vi "Build move command.vi"(8 "error in (no error)":errorcluster, 10 "Command":T1 {"Step style motor 2" items=["", "Single", "Double", "Interleave", "Microstep"]; "Step style motor 1" items=["", "Single", "Double", "Interleave", "Microstep"]; "Direction motor 2" items=["", "Forward", "Backward"]; "Direction motor 1" items=["", "Forward", "Backward"]; "Action" items=["", "Initialize", "Move"]}, 11 "VISA Refnum in":refnum<visa-resource-name>) -> (0 "error out":errorcluster, 2 "String":string, 3 "VISA Refnum out":refnum<visa-resource-name>)   [LabVIEW 2020, in "Arduino-Adafruit stepper.lvlib"]
uses:
  Arduino-Adafruit stepper.lvlib
  Move motor parameters--cluster.ctl
  Motor direction.ctl
  Step style.ctl
  <vilib>/Instr/_visa.llb/VISA Flush IO Buffer Mask.ctl
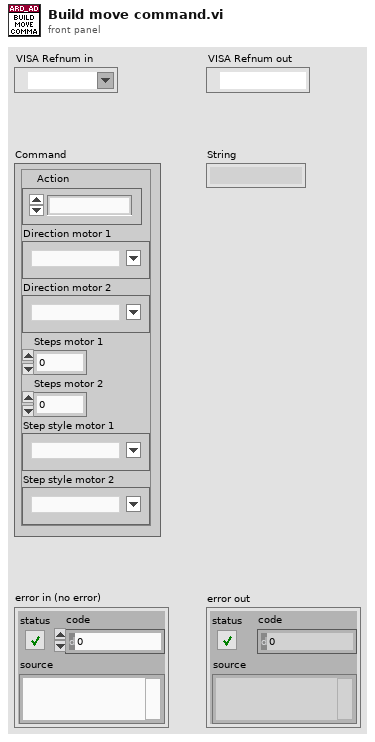
[diagram p1: front panel]
types:
  T1 = typedef "Arduino-Adafruit stepper.lvlib/Move motor parameters--cluster.ctl" = cluster{"Action":u8, "Direction motor 1":T2, "Direction motor 2":T2, "Steps motor 1":u16, "Steps motor 2":u16, "Step style motor 1":T3, "Step style motor 2":T3}
  T2 = typedef "Arduino-Adafruit stepper.lvlib/Motor direction.ctl" = u8
  T3 = typedef "Arduino-Adafruit stepper.lvlib/Step style.ctl" = u8
  T4 = typedef "VISA Flush IO Buffer Mask.ctl" = u16
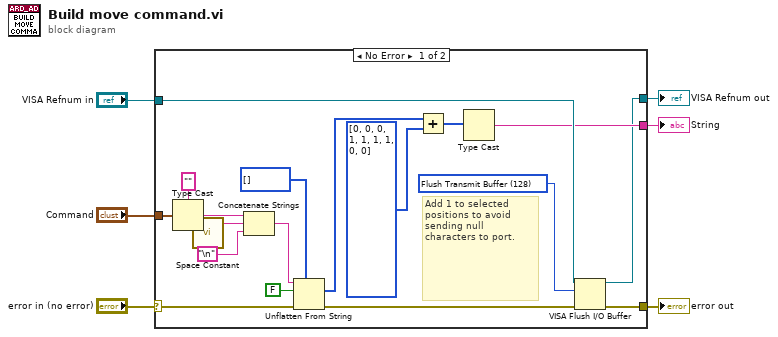
[diagram p0: block diagram]
diagram:
  n1 = case shown="No Error" "error in (no error)" {
    selector: "error in (no error)" -> [w7 w25]
    tunnel: "VISA Refnum in" -> [w24 w26]
    tunnel: [w23 _] -> w5
    tunnel: [w17 w26] -> w4
    tunnel: [w16 w25] -> w3
    tunnel: "Command" -> [w8 _]
    frame No Error {
      w15 = T4 128 items=["Flush Receive Buffer"=16, "Write Transmit Buffer to Device"=32, "Flush Receive Buffer (No I/O)"=64, "Flush Transmit Buffer"=128] ("Mask")
      # "Add 1 to selected positions to avoid sending null characters to port."
      n2 = Type Cast(type="", x=w8) -> (*(type *) &x=w20:string)
      n3 = call <vilib>:"Space Constant.vi"() -> ("String"=w18:string)
      n4 = Concatenate Strings(w20, w18, "\n") -> (w21:string)
      n5 = Unflatten From String(type=u8[] [], binary string=w21, data includes array or string size? (T)=FALSE, error in (no error)=w7) -> (value=w12:u8[], error out=w22:errorcluster)  [unwired: 1 in, 1 out]
      n6 = Add(x=w12, y=u8[] [0, 0, 0, 1, 1, 1, 1, 0, 0]) -> (x+y=w14:u8[])
      n7 = Type Cast(x=w14) -> (*(type *) &x=w23:string)  [unwired: 1 in]
      n8 = VISA Flush I/O Buffer(VISA resource name=w24, mask (16)=w15, error in (no error)=w22) -> (VISA resource name out=w17:refnum<visa-resource-name>, error out=w16:errorcluster)
    }
    frame Error {
    }
  }
  "String" <- w5
  "VISA Refnum out" <- w4
  "error out" <- w3
